vi "Vector Magnitude.vi"(2 "X Component":dbl, 3 "Y Component":dbl) -> (7 "Magnitude":dbl)   [LabVIEW 2012]
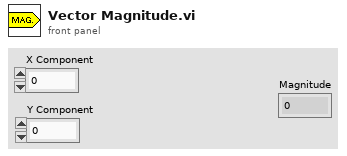
[diagram p1: front panel]
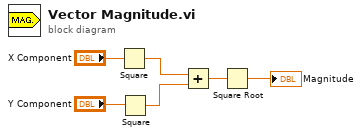
[diagram p0: block diagram]
diagram:
  n1 = Square(x="X Component") -> (x^2=w5:dbl)
  n2 = Square(x="Y Component") -> (x^2=w3:dbl)
  n3 = Add(x=w5, y=w3) -> (x+y=w2:dbl)
  n4 = Square Root(x=w2) -> (sqrt(x)=→"Magnitude":dbl)
